vi "TestNotification.vi"() -> ()   [LabVIEW 2014]
panel:
  in  "stop":bool
  out "error out":errorcluster
  in  "error in (no error)":errorcluster
  in  "path":path
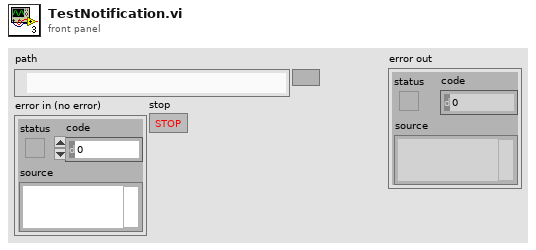
[diagram p1: front panel]
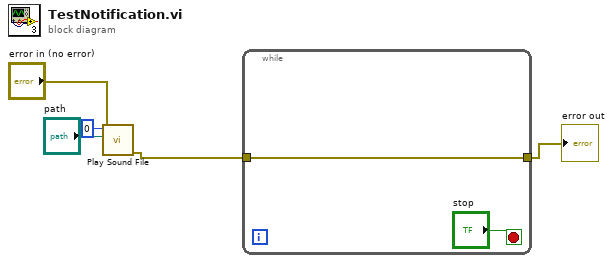
[diagram p0: block diagram]
diagram:
  n1 = call <vilib>:"Play Sound File.vi"("error in (no error)"="error in (no error)", "path"="path", "device ID"=u32 0) -> ("error out"=w2:errorcluster)  [unwired: 7 in, 1 out]
  n2 = while {
    tunnel: w2 -> [w6]
    tunnel: [w6] -> w1
    stop <- "stop" stop-if-true
  }
  "error out" <- w1
